vi "DeserializeInputs.vi"(0 "object in":refnum<class "JSONJKI.lvclass">, 2 "In":variant[](array[variant]), 3 "InputsString":string, 5 "error in (no error)":errorcluster) -> (14 "object out":refnum<class "JSONJKI.lvclass">, 16 "Inputs":variant[](array[variant]), 19 "error out":errorcluster)   [LabVIEW 2018, in "JSONJKI.lvclass"]
uses:
  JSONJKI.lvclass
  <vilib>/addons/_JKI.lib/Serialization/JSON/JKI JSON Serialization.lvlib
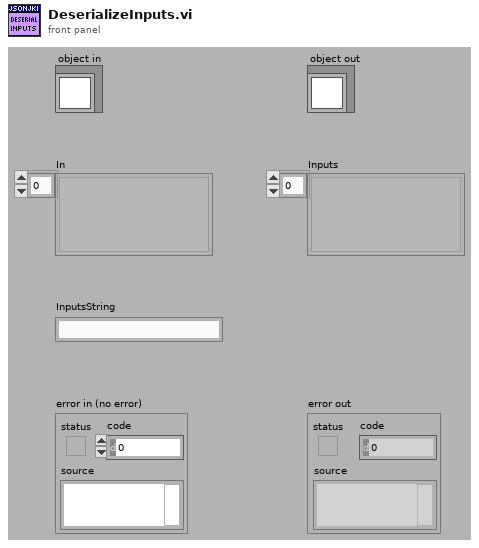
[diagram p1: front panel]
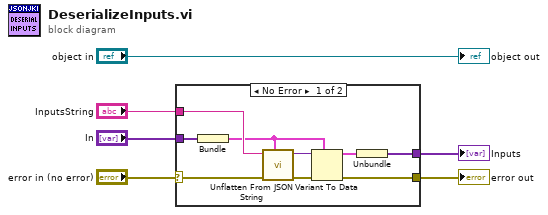
[diagram p0: block diagram]
diagram:
  n1 = case shown="No Error" "error in (no error)" {
    selector: "error in (no error)" -> [w15 w16]
    tunnel: [w14 w16] -> w5
    tunnel: "InputsString" -> [w11 _]
    tunnel: [w13 _] -> w2
    tunnel: "In" -> [w12 _]
    frame No Error {
      n2 = Bundle("In"=w12) -> (w7:cluster{"In":variant[]})  [unwired: 1 in]
      n3 = call <vilib>:"Unflatten From JSON String.vi"("Type and Defaults"=w7, "error in (no error)"=w15, "JSON String"=w11) -> ("error out"=w8:errorcluster, "Variant"=w10:variant)  [unwired: 7 in]
      n4 = Variant To Data(error in=w8, type=w7, Variant=w10) -> (data=w9:cluster{"In":variant[]}, error out=w14:errorcluster)
      n5 = Unbundle(w9) -> ("In"=w13:variant[])
    }
    frame Error {
    }
  }
  "error out" <- w5
  "Inputs" <- w2
  "object out" <- "object in"
